vi "SingleObject.vi"(8 "error in (no error)":errorcluster) -> (0 "error out":errorcluster, 3 "Instance out":refnum<data-value>)   [LabVIEW 2018, in "SingleObject.lvclass"]
uses:
  SingleObject.lvclass
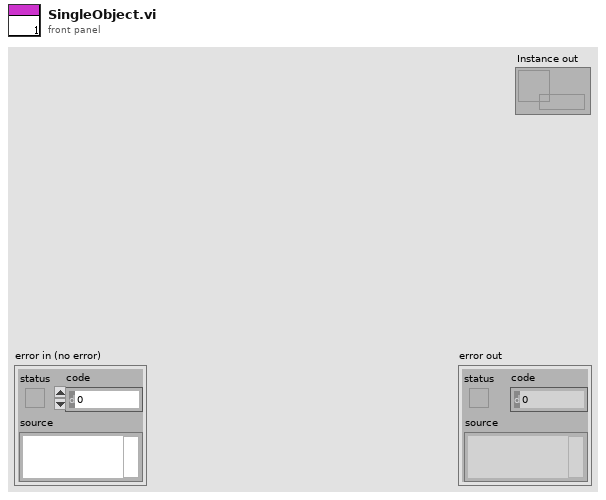
[diagram p1: front panel]
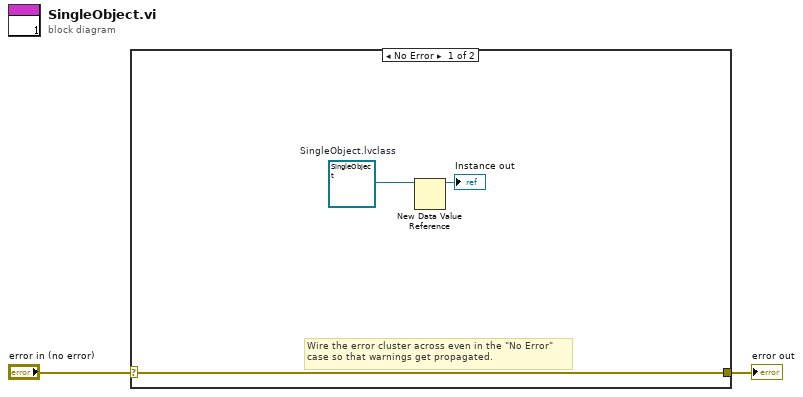
[diagram p0: block diagram]
diagram:
  n1 = case shown="No Error" "error in (no error)" {
    selector: "error in (no error)" -> [w5 w6]
    tunnel: [w5 w6] -> w1
    frame No Error {
      w4 = refnum<class "SingleObject.lvclass"> refnum  # SingleObject.lvclass
      # "Wire the error cluster across even in the \"No Error\"\ncase so that warnings get propagated."
      n2 = New Data Value Reference(data value=w4) -> (data value reference=→"Instance out":refnum<data-value>)  [unwired: 1 in, 1 out]
    }
    frame Error {
    }
  }
  "error out" <- w1
